vi "ParseSubUIs.vi"(10 "Arguments":string, 11 "UIs":T1) -> (3 "UI_DAQ_config out":refnum<class "UI_DAQ_config.lvclass">)   [LabVIEW 2016, in "UI_Main.lvclass"]
uses:
  UI_Main.lvclass
  UI_DAQ_config/UI_DAQ_config.lvclass
  Typedefs/SubUIs.ctl
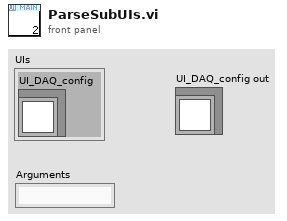
[diagram p1: front panel]
types:
  T1 = typedef "UI_Main.lvclass/SubUIs.ctl" = cluster{"UI_DAQ_config":refnum<class "UI_DAQ_config.lvclass">}
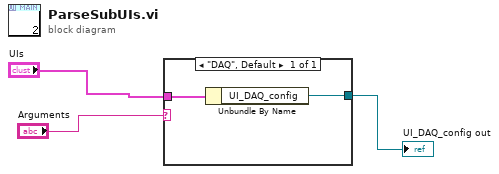
[diagram p0: block diagram]
diagram:
  n1 = case shown="\"DAQ\", Default" "Arguments" {
    tunnel: [w5] -> w2
    tunnel: "UIs" -> [w4]
    frame "DAQ", Default {
      n2 = Unbundle By Name(w4) -> ("UI_DAQ_config"=w5:refnum<class "UI_DAQ_config.lvclass">)
    }
  }
  "UI_DAQ_config out" <- w2
